vi "libssh2_agent_set_identity_path.vi"(8 "error in (no error)":errorcluster, 10 "path":path, 11 "agent":T1) -> (0 "error out":errorcluster)   [LabVIEW 2013, in "libssh2.lvlib"]
doc: "Set the path to a custom identity socket instead of the default <B>SSH_AUTH_SOCK</B> environment variable."
uses:
  libssh2.lvlib
  Agent Refnum.ctl
  Not An Agent.vi
  <vilib>/Utility/error.llb/Error Cluster From Error Code.vi
  Global Settings.vi
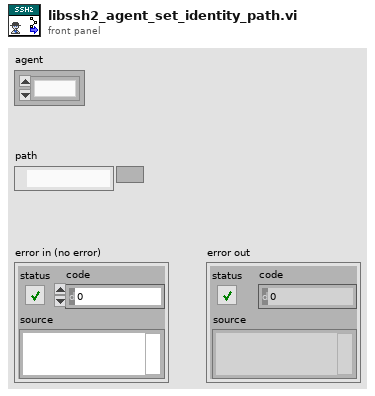
[diagram p1: front panel]
types:
  T1 = typedef "libssh2.lvlib/Agent Refnum.ctl" = refnum<k1>
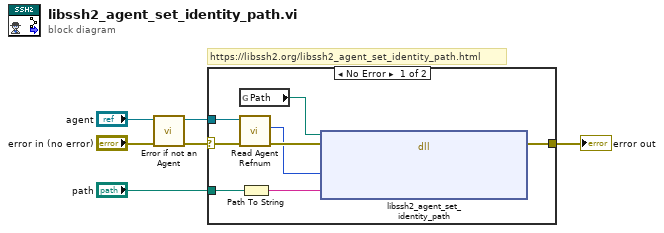
[diagram p0: block diagram]
diagram:
  # "https://libssh2.org/libssh2_agent_set_identity_path.html"
  n1 = call "Error if not an Agent.vi"("error in (no error)"="error in (no error)", "agent"="agent") -> ("error out"=w3:errorcluster, "agent out"=w1:T1)  [unwired: 8 in]
  n2 = case shown="No Error" w3 {
    selector: w3 -> [w14 w15]
    tunnel: [w7 w15] -> w6
    tunnel: w1 -> [w13 _]
    tunnel: "path" -> [w12 _]
    frame No Error {
      n3 = global read "Global Settings.vi" "Path"() -> (w11:path)
      n4 = call "Read Agent Refnum.vi"("error in (no error)"=w14, "agent"=w13) -> ("error out"=w10:errorcluster, "LIBSSH2_AGENT*"=w9:u64)  [unwired: 8 in]
      n5 = Path To String(path=w12) -> (string=w8:string)
      n6 = dll-call lib="?" fn="libssh2_agent_set_identity_path"(path in=w11, error in=w10, "agent"=w9, "path"=w8) -> (error out=w7:errorcluster)  [unwired: 4 in, 1 out]
    }
    frame Error {
    }
  }
  "error out" <- w6
